vi "Is Data Ready.vi"(8 "error in (no error)":errorcluster, 11 "DAQmx Digitizer in":refnum<class "DAQmx Digitizer.lvclass">) -> (0 "error out":errorcluster, 1 "Data ready":bool, 2 "Availiable Samples":u32, 3 "DAQmx Digitizer out":refnum<class "DAQmx Digitizer.lvclass">)   [LabVIEW 2015, in "DAQmx Digitizer.lvclass"]
uses:
  DAQmx Digitizer.lvclass
  Instruments/Pulse Driver/Pulse Driver.lvclass/Pulse Driver.ctl
  DAQmx Digitizer.lvclass/DAQmx Digitizer.ctl
  Instruments/Pulse Driver/Read Samples per read.vi
  Instruments/Pulse Driver/Read Samples per channel.vi
  <resource>/objmgr/daqmx.rc
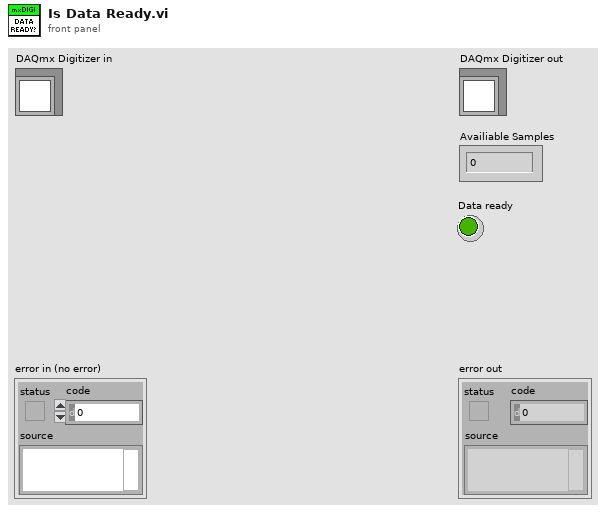
[diagram p1: front panel]
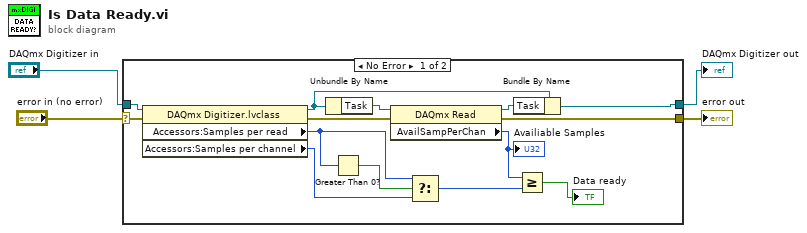
[diagram p0: block diagram]
diagram:
  n1 = case shown="No Error" "error in (no error)" {
    selector: "error in (no error)" -> [w6 w20]
    tunnel: [w17 w20] -> w2
    tunnel: [w16 w19] -> w1
    tunnel: "DAQmx Digitizer in" -> [w18 w19]
    frame No Error {
      n2 = property class="DAQmx Digitizer.lvclass"(reference=w18, error in=w6) -> (reference out=w11:refnum<class "DAQmx Digitizer.lvclass">, error out=w5:errorcluster, "Accessors:Samples per read"=w9:i32, "Accessors:Samples per channel"=w8:i32)
      n3 = Unbundle By Name(w11) -> ("Task"=w12:refnum<k21>)
      n4 = Greater Than 0?(x=w9) -> (x > 0?=w10:bool)
      n5 = property class="DAQmx Read"(reference=w12, error in=w5) -> (reference out=w15:refnum<k21>, error out=w17:errorcluster, "AvailSampPerChan"=w14:u32)
      "Availiable Samples" <- w14
      n6 = Select(t=w9, s=w10, f=w8) -> (s? t:f=w7:i32)
      n7 = Bundle By Name(cluster=w11, "Task"=w15) -> (w16:refnum<class "DAQmx Digitizer.lvclass">)
      n8 = Greater Or Equal?(x=w14, y=w7) -> (x >= y?=→"Data ready":bool)
    }
    frame Error {
    }
  }
  "error out" <- w2
  "DAQmx Digitizer out" <- w1
